vi "enumerateStaticDependencies.vi"(8 "error in (no error)":errorcluster, 11 "SMO":refnum<class "SMO.lvclass">) -> (0 "error out":errorcluster, 2 "Static Dependencies":refnum<class "SMODependency.lvclass">[](array[class]), 3 "SMO out":refnum<class "SMO.lvclass">)   [LabVIEW 2013, in "SMO.lvclass"]
uses:
  SMO.lvclass
  Dependency/SMODependency.lvclass
panel:
  # "For instructions on how to use the JKI State Machine Objects, examples and video tutorials, visit:\nhttp://jki.net/state-machine-objects/\n\nJKI State Machine Objects™\nhttp://jki.net/state-machine-objects/\nCopyright (C) 2005-2015, JKI <info@jki.net>\nALL RIGHTS RESERVED"
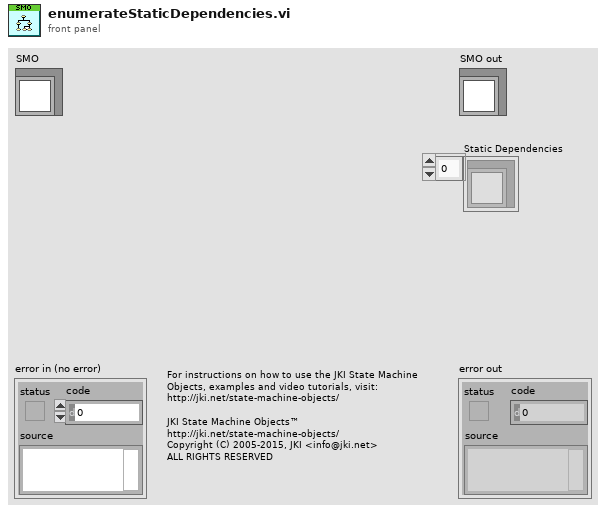
[diagram p1: front panel]
types:
  T1 = cluster{"First":refnum<class "SMO.lvclass">, "Second":refnum<class "SMO.lvclass">}
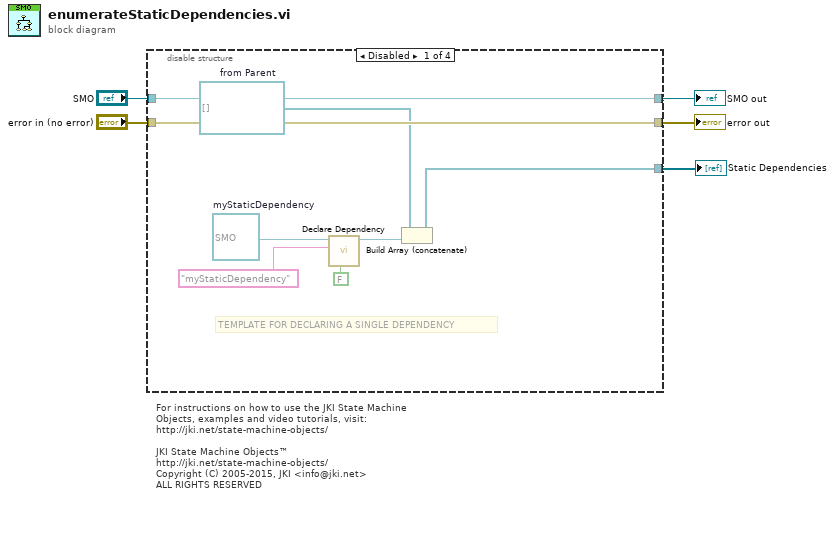
[diagram p0: block diagram]
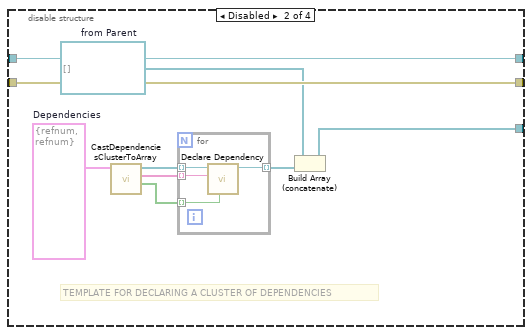
[diagram p2: hidden frame]
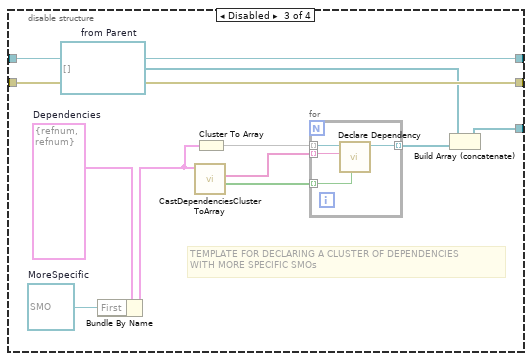
[diagram p3: hidden frame]
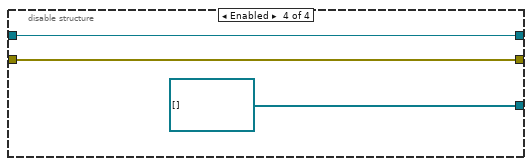
[diagram p4: hidden frame]
diagram:
  # "For instructions on how to use the JKI State Machine Objects, examples and video tutorials, visit:\nhttp://jki.net/state-machine-objects/\n\nJKI State Machine Objects™\nhttp://jki.net/state-machine-objects/\nCopyright (C) 2005-2015, JKI <info@jki.net>\nALL RIGHTS RESERVED"
  n1 = disable-structure shown="Disabled" {
    disable-tunnel: "SMO" -> [w13 w22 w37 w44]
    disable-tunnel: [w13 w22 w37 w44] -> w4
    disable-tunnel: "error in (no error)" -> [w12 w21 w36 w43]
    disable-tunnel: [w12 w21 w36 w43] -> w2
    disable-tunnel: [w7 w19 w34 refnum<class "SMODependency.lvclass">[] [] ("appended array")] -> w1
    frame Disabled {
      w6 = refnum<class "SMODependency.lvclass">[] []  # from Parent
      w11 = refnum<class "SMO.lvclass"> refnum  # myStaticDependency
      # "TEMPLATE FOR DECLARING A SINGLE DEPENDENCY"
      n2 = call "Declare Dependency.vi"("Shared Resource (F)"=FALSE, "Name"="myStaticDependency", "Type"=w11) -> ("SMODependency out"=w8:refnum<class "SMODependency.lvclass">)  [unwired: 7 in, 1 out]
      n3 = Build Array (concatenate)(w6, w8) -> (w7:refnum<class "SMODependency.lvclass">[])
    }
    frame Disabled {
      w17 = T1 {"First"=refnum, "Second"=refnum}  # Dependencies
      w18 = refnum<class "SMODependency.lvclass">[] []  # from Parent
      # "TEMPLATE FOR DECLARING A CLUSTER OF DEPENDENCIES"
      n4 = call "CastDependenciesClusterToArray.vi"("Dependencies Cluster"=w17) -> ("Shared Resources"=w14:bool[], "Dependencies Names"=w15:string[], "Dependencies Array"=w16:refnum<class "SMO.lvclass">[])  [unwired: 8 in]
      n5 = for {
        tunnel: [w26] -> w20 mode=indexing
        tunnel: w16 -> [w25] mode=indexing
        tunnel: w15 -> [w24] mode=indexing
        tunnel: w14 -> [w23] mode=indexing
        n6 = call "Declare Dependency.vi"("Shared Resource (F)"=w23, "Name"=w24, "Type"=w25) -> ("SMODependency out"=w26:refnum<class "SMODependency.lvclass">)  [unwired: 7 in, 1 out]
      }
      n7 = Build Array (concatenate)(w18, w20) -> (w19:refnum<class "SMODependency.lvclass">[])
    }
    frame Disabled {
      w29 = refnum<class "SMO.lvclass"> refnum  # MoreSpecific
      w30 = T1 {"First"=refnum, "Second"=refnum}  # Dependencies
      w33 = refnum<class "SMODependency.lvclass">[] []  # from Parent
      # "TEMPLATE FOR DECLARING A CLUSTER OF DEPENDENCIES\nWITH MORE SPECIFIC SMOs"
      n8 = Bundle By Name(cluster=w30, "First"=w29) -> (w27:T1)
      n9 = call "CastDependenciesClusterToArray.vi"("Dependencies Cluster"=w27) -> ("Shared Resources"=w31:bool[], "Dependencies Names"=w32:string[])  [unwired: 8 in, 1 out]
      n10 = Cluster To Array(cluster=w27) -> (array=w28:refnum<class "SMO.lvclass">[])
      n11 = for {
        tunnel: [w41] -> w35 mode=indexing
        tunnel: w28 -> [w40] mode=indexing
        tunnel: w32 -> [w39] mode=indexing
        tunnel: w31 -> [w38] mode=indexing
        n12 = call "Declare Dependency.vi"("Shared Resource (F)"=w38, "Name"=w39, "Type"=w40) -> ("SMODependency out"=w41:refnum<class "SMODependency.lvclass">)  [unwired: 7 in, 1 out]
      }
      n13 = Build Array (concatenate)(w33, w35) -> (w34:refnum<class "SMODependency.lvclass">[])
    }
    frame Enabled {
    }
  }
  "error out" <- w2
  "SMO out" <- w4
  "Static Dependencies" <- w1
